vi "Abadines_Server2.vi"() -> ()   [LabVIEW 2013]
uses:
  <vilib>/NXT/Block Support/NXT_MessageMailbox.ctl
  <vilib>/NXT/Block Support/NXT_InputPort.ctl
  <vilib>/NXT/Dual Mode Library/BT/BlueTooth_Write_Num.vi
  <vilib>/NXT/Subs/MotorOutput.ctl
  <vilib>/NXT/Block Support/NXT_OutputPort.ctl
  <vilib>/NXT/LegoClasses/BrickReference/BrickReference.lvclass
  <vilib>/NXT/Subs/LVHSConnector.ctl
  <vilib>/NXT/NXTIO Xnodes/NXTIONodeSubVIs/NXTStopMotors.vi
  <vilib>/NXT/NXTIO Xnodes/NXTIOXNode/NXTIO.xnode
  <vilib>/NXT/NXTIO Xnodes/AddressXNode/NXTIOAddress.xnode
  <vilib>/NXT/Dual Mode Library/Sound/PlayRedPianoFile.vi
panel:
  out "Blue Line":i16
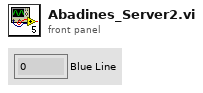
[diagram p1: front panel]
types:
  T1 = typedef "LVHSConnector.ctl" = refnum<class "BrickReference.lvclass">
  T2 = typedef "NXT_InputPort.ctl" = u32
  T3 = typedef "NXT_MessageMailbox.ctl" = u8
  T4 = typedef "NXT_OutputPort.ctl" = u8
  T5 = typedef "MotorOutput.ctl" = u8
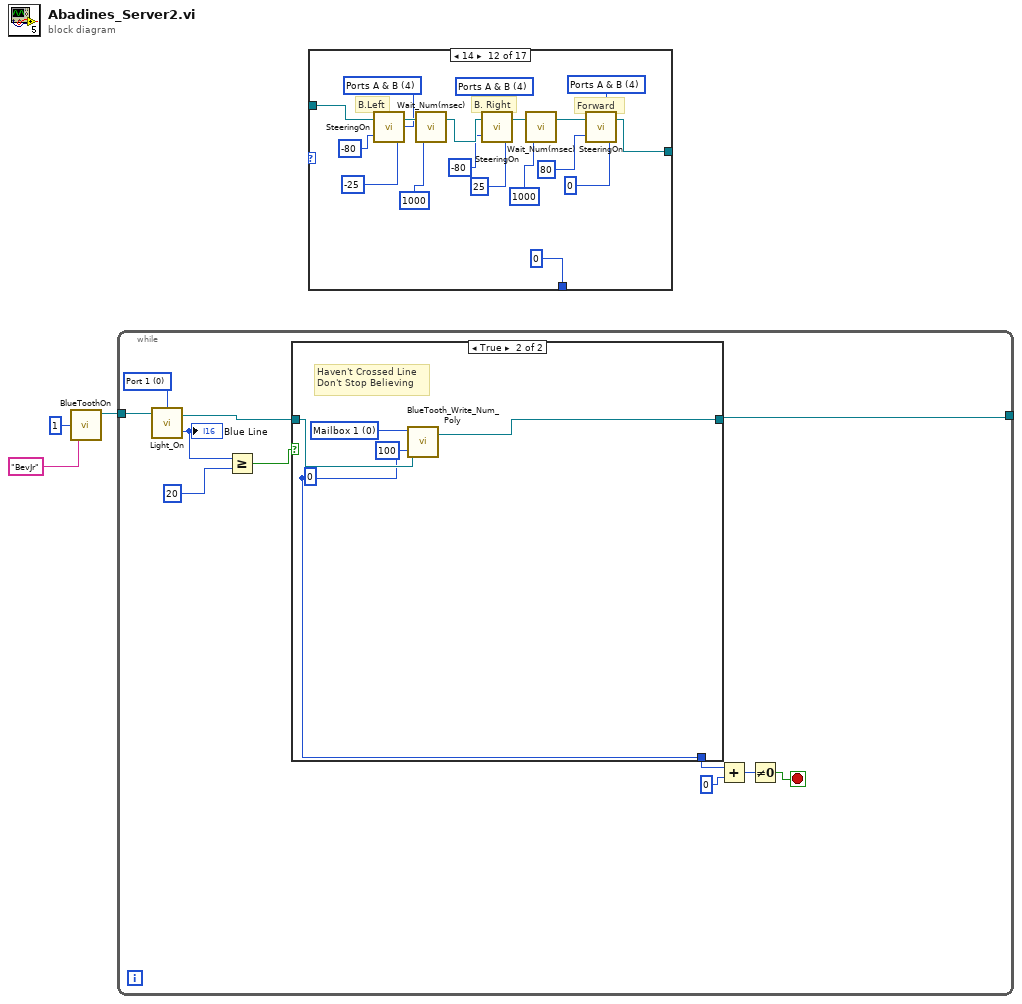
[diagram p0: block diagram]
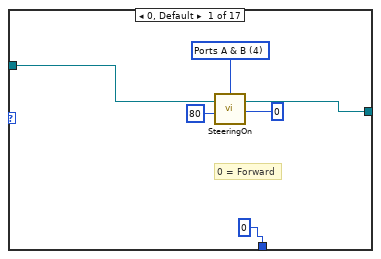
[diagram p2: hidden frame]
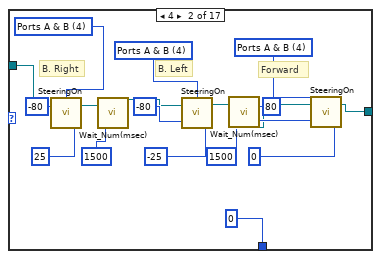
[diagram p3: hidden frame]
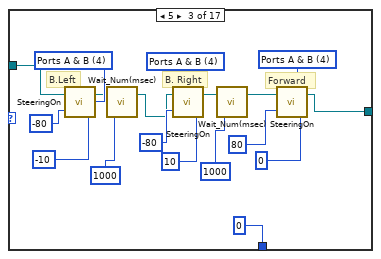
[diagram p4: hidden frame]
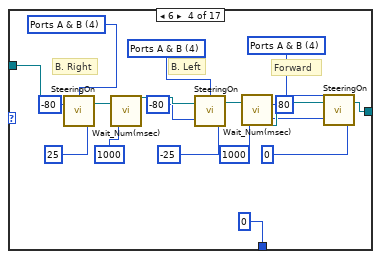
[diagram p5: hidden frame]
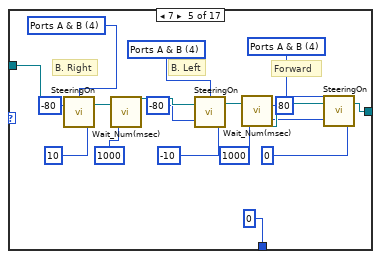
[diagram p6: hidden frame]
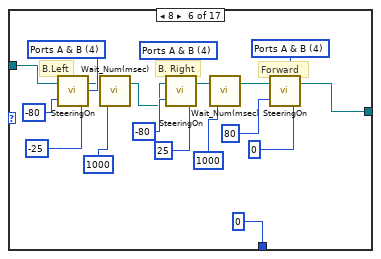
[diagram p7: hidden frame]
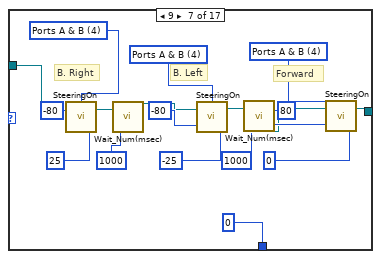
[diagram p8: hidden frame]
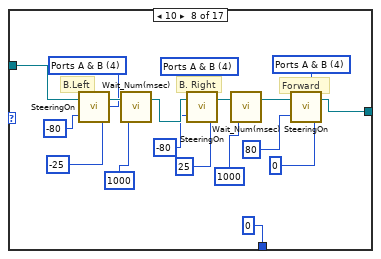
[diagram p9: hidden frame]
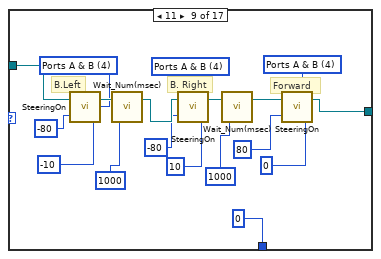
[diagram p10: hidden frame]
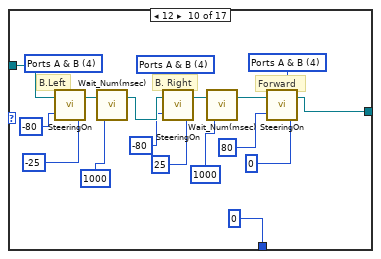
[diagram p11: hidden frame]
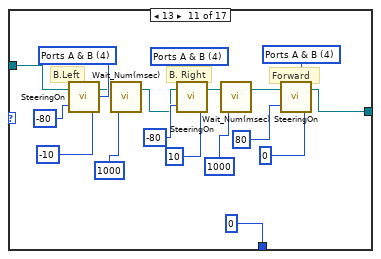
[diagram p12: hidden frame]
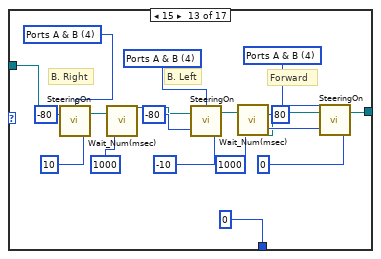
[diagram p13: hidden frame]
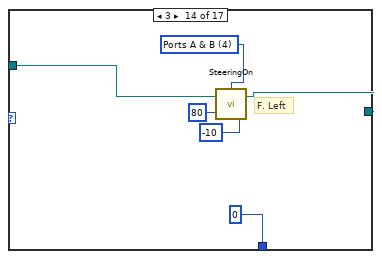
[diagram p14: hidden frame]
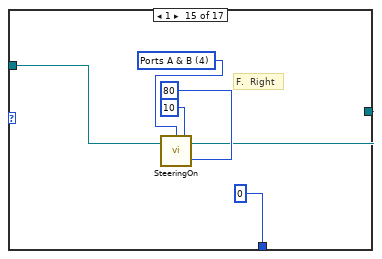
[diagram p15: hidden frame]
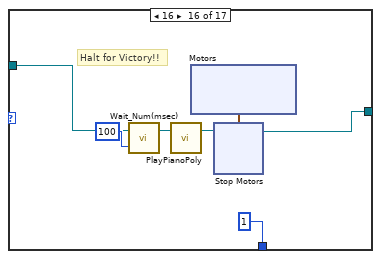
[diagram p16: hidden frame]
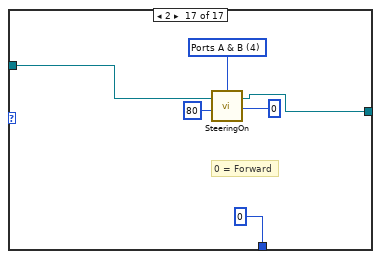
[diagram p17: hidden frame]
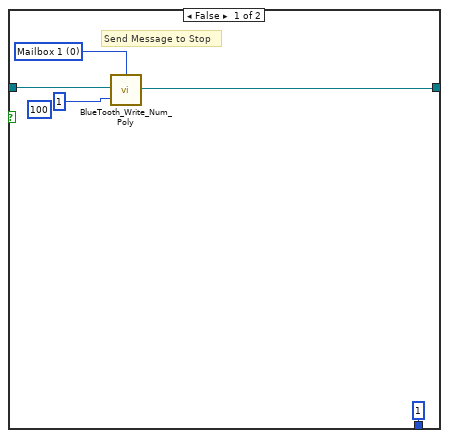
[diagram p18: hidden frame]
diagram:
  n1 = call "BlueToothOn.vi"("Connection"=u8 1, "Partner Name"="BevJr") -> ("NXT/EV3 2"=w2:T1)  [unwired: 1 in, 3 out]
  n2 = while {
    tunnel: w2 -> [w15]
    tunnel: [w9] -> _
    stop <- w5 stop-if-true
    w14 = T2 0 items=["Port 1", "Port 2", "Port 3", "Port 4"] ("Port (Port 3)")
    n3 = call <vilib>:"Light_On.vi"("NXT/EV3"=w15, "Port (Port 3)"=w14) -> ("Scaled Value"=w13:i16, "NXT/EV3"=w10:T1)  [unwired: 1 in]
    "Blue Line" <- w13
    n4 = Greater Or Equal?(x=w13, y=i16 20) -> (x >= y?=w11:bool)
    n5 = case shown="True" w11 {
      tunnel: w10 -> [w18 w23]
      tunnel: [w16 w22] -> w9
      tunnel: [1 w21] -> w8
      frame False {
        (unwired) u16 100 ("Tone (440 Hz)")
        w19 = T3 0 items=["Mailbox 1", "Mailbox 2", "Mailbox 3", "Mailbox 4", "Mailbox 5", "Mailbox 6", "Mailbox 7", "Mailbox 8", "Mailbox 9", "Mailbox 10"] ("Mailbox")
        # "Send Message to Stop"
        n6 = call-poly <vilib>:"BlueTooth_Write_Num_Poly.vi"("Message"=1, "NXT/EV3"=w18, "Mailbox"=w19) -> ("NXT/EV3"=w16:T1)  [unwired: 1 in]
      }
      frame True {
        (unwired) u16 100 ("Tone (440 Hz)")
        w24 = T3 0 items=["Mailbox 1", "Mailbox 2", "Mailbox 3", "Mailbox 4", "Mailbox 5", "Mailbox 6", "Mailbox 7", "Mailbox 8", "Mailbox 9", "Mailbox 10"] ("Mailbox")
        w21 = 0 ("Message")
        # "Haven't Crossed Line\nDon't Stop Believing"
        n7 = call-poly <vilib>:"BlueTooth_Write_Num_Poly.vi"("Message"=w21, "NXT/EV3"=w23, "Mailbox"=w24) -> ("NXT/EV3"=w22:T1)  [unwired: 1 in]
      }
    }
    n8 = Add(x=w8, y=0) -> (x+y=w6:i32)
    n9 = Not Equal To 0?(x=w6) -> (x != 0?=w5:bool)
  }
  n10 = case shown="14" {
    selector: _ -> [_ _ _ _ _ _ _ _ _ _ _ _ _ _ _ _ _]
    tunnel: _ -> [w28 w42 w51 w69 w87 w114 w123 w141 w159 w177 w194 w212 w231 w249 w255 w260 w274]
    tunnel: [w27 w41 w50 w68 w86 w113 w122 w140 w158 w176 w193 w211 w230 w248 w254 w261 w273] -> w1
    tunnel: [0 ("y") 0 ("y") 0 ("y") 0 ("y") 0 ("y") 0 ("y") 0 ("y") 0 ("y") 0 ("y") 0 ("y") 0 ("y") 0 ("y") 0 ("y") 0 ("y") 0 1 0 ("y")] -> _
    frame 0, Default {
      w26 = T5 4 items=["Port A"=0, "Port B"=1, "Port C"=2, "Ports A & B"=4, "Ports A & C"=5, "Ports B & C"=6, "All Ports"=3] ("Output Ports (A & B) 5")
      # "0 = Forward"
      n11 = call <vilib>:"SteeringOn.vi"("Power (75)"=80, "Steering (100)"=0, "NXT/EV3"=w28, "Output Ports (A & B)"=w26) -> ("NXT/EV3"=w27:T1)
    }
    frame 4 {
      w38 = T5 4 items=["Port A"=0, "Port B"=1, "Port C"=2, "Ports A & B"=4, "Ports A & C"=5, "Ports B & C"=6, "All Ports"=3] ("Output Ports (A & B) 15")
      w39 = T5 4 items=["Port A"=0, "Port B"=1, "Port C"=2, "Ports A & B"=4, "Ports A & C"=5, "Ports B & C"=6, "All Ports"=3] ("Output Port (All Ports) 6")
      w40 = T5 4 items=["Port A"=0, "Port B"=1, "Port C"=2, "Ports A & B"=4, "Ports A & C"=5, "Ports B & C"=6, "All Ports"=3] ("Output Ports (A & B) 16")
      # "Forward"
      # "B. Left"
      # "B. Right"
      n12 = call <vilib>:"SteeringOn.vi"("Power (75)"=-80, "Steering (100)"=25, "NXT/EV3"=w42, "Output Ports (A & B)"=w40) -> ("NXT/EV3"=w37:T1)
      n13 = call <vilib>:"Wait_Num(msec).vi"("Time (100 msec)"=u32 1500, "NXT/EV3"=w37) -> ("NXT/EV3"=w36:T1)  [unwired: 2 in]
      n14 = call <vilib>:"SteeringOn.vi"("Power (75)"=-80, "Steering (100)"=-25, "NXT/EV3"=w36, "Output Ports (A & B)"=w39) -> ("NXT/EV3"=w35:T1)
      n15 = call <vilib>:"Wait_Num(msec).vi"("Time (100 msec)"=u32 1500, "NXT/EV3"=w35) -> ("NXT/EV3"=w34:T1)  [unwired: 2 in]
      n16 = call <vilib>:"SteeringOn.vi"("Power (75)"=80, "Steering (100)"=0, "NXT/EV3"=w34, "Output Ports (A & B)"=w38) -> ("NXT/EV3"=w41:T1)
    }
    frame 5 {
      w58 = T5 4 items=["Port A"=0, "Port B"=1, "Port C"=2, "Ports A & B"=4, "Ports A & C"=5, "Ports B & C"=6, "All Ports"=3] ("Output Ports (A & B) 21")
      w59 = T5 4 items=["Port A"=0, "Port B"=1, "Port C"=2, "Ports A & B"=4, "Ports A & C"=5, "Ports B & C"=6, "All Ports"=3] ("Output Port (All Ports) 9")
      w60 = T5 4 items=["Port A"=0, "Port B"=1, "Port C"=2, "Ports A & B"=4, "Ports A & C"=5, "Ports B & C"=6, "All Ports"=3] ("Output Ports (A & B) 22")
      # "Forward"
      # "B. Right"
      # "B.Left"
      n17 = call <vilib>:"SteeringOn.vi"("Power (75)"=-80, "Steering (100)"=-10, "NXT/EV3"=w51, "Output Ports (A & B)"=w60) -> ("NXT/EV3"=w56:T1)
      n18 = call <vilib>:"Wait_Num(msec).vi"("Time (100 msec)"=u32 1000, "NXT/EV3"=w56) -> ("NXT/EV3"=w55:T1)  [unwired: 2 in]
      n19 = call <vilib>:"SteeringOn.vi"("Power (75)"=-80, "Steering (100)"=10, "NXT/EV3"=w55, "Output Ports (A & B)"=w59) -> ("NXT/EV3"=w53:T1)
      n20 = call <vilib>:"Wait_Num(msec).vi"("Time (100 msec)"=u32 1000, "NXT/EV3"=w53) -> ("NXT/EV3"=w52:T1)  [unwired: 2 in]
      n21 = call <vilib>:"SteeringOn.vi"("Power (75)"=80, "Steering (100)"=0, "NXT/EV3"=w52, "Output Ports (A & B)"=w58) -> ("NXT/EV3"=w50:T1)
    }
    frame 6 {
      w78 = T5 4 items=["Port A"=0, "Port B"=1, "Port C"=2, "Ports A & B"=4, "Ports A & C"=5, "Ports B & C"=6, "All Ports"=3] ("Output Ports (A & B) 15")
      w77 = T5 4 items=["Port A"=0, "Port B"=1, "Port C"=2, "Ports A & B"=4, "Ports A & C"=5, "Ports B & C"=6, "All Ports"=3] ("Output Port (All Ports) 6")
      w76 = T5 4 items=["Port A"=0, "Port B"=1, "Port C"=2, "Ports A & B"=4, "Ports A & C"=5, "Ports B & C"=6, "All Ports"=3] ("Output Ports (A & B) 16")
      # "Forward"
      # "B. Left"
      # "B. Right"
      n22 = call <vilib>:"SteeringOn.vi"("Power (75)"=-80, "Steering (100)"=25, "NXT/EV3"=w69, "Output Ports (A & B)"=w76) -> ("NXT/EV3"=w79:T1)
      n23 = call <vilib>:"Wait_Num(msec).vi"("Time (100 msec)"=u32 1000, "NXT/EV3"=w79) -> ("NXT/EV3"=w80:T1)  [unwired: 2 in]
      n24 = call <vilib>:"SteeringOn.vi"("Power (75)"=-80, "Steering (100)"=-25, "NXT/EV3"=w80, "Output Ports (A & B)"=w77) -> ("NXT/EV3"=w81:T1)
      n25 = call <vilib>:"Wait_Num(msec).vi"("Time (100 msec)"=u32 1000, "NXT/EV3"=w81) -> ("NXT/EV3"=w82:T1)  [unwired: 2 in]
      n26 = call <vilib>:"SteeringOn.vi"("Power (75)"=80, "Steering (100)"=0, "NXT/EV3"=w82, "Output Ports (A & B)"=w78) -> ("NXT/EV3"=w68:T1)
    }
    frame 7 {
      w96 = T5 4 items=["Port A"=0, "Port B"=1, "Port C"=2, "Ports A & B"=4, "Ports A & C"=5, "Ports B & C"=6, "All Ports"=3] ("Output Ports (A & B) 15")
      w95 = T5 4 items=["Port A"=0, "Port B"=1, "Port C"=2, "Ports A & B"=4, "Ports A & C"=5, "Ports B & C"=6, "All Ports"=3] ("Output Port (All Ports) 6")
      w94 = T5 4 items=["Port A"=0, "Port B"=1, "Port C"=2, "Ports A & B"=4, "Ports A & C"=5, "Ports B & C"=6, "All Ports"=3] ("Output Ports (A & B) 16")
      # "Forward"
      # "B. Left"
      # "B. Right"
      n27 = call <vilib>:"SteeringOn.vi"("Power (75)"=-80, "Steering (100)"=10, "NXT/EV3"=w87, "Output Ports (A & B)"=w94) -> ("NXT/EV3"=w97:T1)
      n28 = call <vilib>:"Wait_Num(msec).vi"("Time (100 msec)"=u32 1000, "NXT/EV3"=w97) -> ("NXT/EV3"=w98:T1)  [unwired: 2 in]
      n29 = call <vilib>:"SteeringOn.vi"("Power (75)"=-80, "Steering (100)"=-10, "NXT/EV3"=w98, "Output Ports (A & B)"=w95) -> ("NXT/EV3"=w99:T1)
      n30 = call <vilib>:"Wait_Num(msec).vi"("Time (100 msec)"=u32 1000, "NXT/EV3"=w99) -> ("NXT/EV3"=w100:T1)  [unwired: 2 in]
      n31 = call <vilib>:"SteeringOn.vi"("Power (75)"=80, "Steering (100)"=0, "NXT/EV3"=w100, "Output Ports (A & B)"=w96) -> ("NXT/EV3"=w86:T1)
    }
    frame 8 {
      w110 = T5 4 items=["Port A"=0, "Port B"=1, "Port C"=2, "Ports A & B"=4, "Ports A & C"=5, "Ports B & C"=6, "All Ports"=3] ("Output Ports (A & B) 21")
      w111 = T5 4 items=["Port A"=0, "Port B"=1, "Port C"=2, "Ports A & B"=4, "Ports A & C"=5, "Ports B & C"=6, "All Ports"=3] ("Output Port (All Ports) 9")
      w112 = T5 4 items=["Port A"=0, "Port B"=1, "Port C"=2, "Ports A & B"=4, "Ports A & C"=5, "Ports B & C"=6, "All Ports"=3] ("Output Ports (A & B) 22")
      # "Forward"
      # "B. Right"
      # "B.Left"
      n32 = call <vilib>:"SteeringOn.vi"("Power (75)"=-80, "Steering (100)"=-25, "NXT/EV3"=w114, "Output Ports (A & B)"=w112) -> ("NXT/EV3"=w108:T1)
      n33 = call <vilib>:"Wait_Num(msec).vi"("Time (100 msec)"=u32 1000, "NXT/EV3"=w108) -> ("NXT/EV3"=w107:T1)  [unwired: 2 in]
      n34 = call <vilib>:"SteeringOn.vi"("Power (75)"=-80, "Steering (100)"=25, "NXT/EV3"=w107, "Output Ports (A & B)"=w111) -> ("NXT/EV3"=w105:T1)
      n35 = call <vilib>:"Wait_Num(msec).vi"("Time (100 msec)"=u32 1000, "NXT/EV3"=w105) -> ("NXT/EV3"=w104:T1)  [unwired: 2 in]
      n36 = call <vilib>:"SteeringOn.vi"("Power (75)"=80, "Steering (100)"=0, "NXT/EV3"=w104, "Output Ports (A & B)"=w110) -> ("NXT/EV3"=w113:T1)
    }
    frame 9 {
      w130 = T5 4 items=["Port A"=0, "Port B"=1, "Port C"=2, "Ports A & B"=4, "Ports A & C"=5, "Ports B & C"=6, "All Ports"=3] ("Output Ports (A & B) 15")
      w131 = T5 4 items=["Port A"=0, "Port B"=1, "Port C"=2, "Ports A & B"=4, "Ports A & C"=5, "Ports B & C"=6, "All Ports"=3] ("Output Port (All Ports) 6")
      w132 = T5 4 items=["Port A"=0, "Port B"=1, "Port C"=2, "Ports A & B"=4, "Ports A & C"=5, "Ports B & C"=6, "All Ports"=3] ("Output Ports (A & B) 16")
      # "Forward"
      # "B. Left"
      # "B. Right"
      n37 = call <vilib>:"SteeringOn.vi"("Power (75)"=-80, "Steering (100)"=25, "NXT/EV3"=w123, "Output Ports (A & B)"=w132) -> ("NXT/EV3"=w129:T1)
      n38 = call <vilib>:"Wait_Num(msec).vi"("Time (100 msec)"=u32 1000, "NXT/EV3"=w129) -> ("NXT/EV3"=w128:T1)  [unwired: 2 in]
      n39 = call <vilib>:"SteeringOn.vi"("Power (75)"=-80, "Steering (100)"=-25, "NXT/EV3"=w128, "Output Ports (A & B)"=w131) -> ("NXT/EV3"=w127:T1)
      n40 = call <vilib>:"Wait_Num(msec).vi"("Time (100 msec)"=u32 1000, "NXT/EV3"=w127) -> ("NXT/EV3"=w126:T1)  [unwired: 2 in]
      n41 = call <vilib>:"SteeringOn.vi"("Power (75)"=80, "Steering (100)"=0, "NXT/EV3"=w126, "Output Ports (A & B)"=w130) -> ("NXT/EV3"=w122:T1)
    }
    frame 10 {
      w150 = T5 4 items=["Port A"=0, "Port B"=1, "Port C"=2, "Ports A & B"=4, "Ports A & C"=5, "Ports B & C"=6, "All Ports"=3] ("Output Ports (A & B) 21")
      w149 = T5 4 items=["Port A"=0, "Port B"=1, "Port C"=2, "Ports A & B"=4, "Ports A & C"=5, "Ports B & C"=6, "All Ports"=3] ("Output Port (All Ports) 9")
      w148 = T5 4 items=["Port A"=0, "Port B"=1, "Port C"=2, "Ports A & B"=4, "Ports A & C"=5, "Ports B & C"=6, "All Ports"=3] ("Output Ports (A & B) 22")
      # "Forward"
      # "B. Right"
      # "B.Left"
      n42 = call <vilib>:"SteeringOn.vi"("Power (75)"=-80, "Steering (100)"=-25, "NXT/EV3"=w141, "Output Ports (A & B)"=w148) -> ("NXT/EV3"=w152:T1)
      n43 = call <vilib>:"Wait_Num(msec).vi"("Time (100 msec)"=u32 1000, "NXT/EV3"=w152) -> ("NXT/EV3"=w153:T1)  [unwired: 2 in]
      n44 = call <vilib>:"SteeringOn.vi"("Power (75)"=-80, "Steering (100)"=25, "NXT/EV3"=w153, "Output Ports (A & B)"=w149) -> ("NXT/EV3"=w155:T1)
      n45 = call <vilib>:"Wait_Num(msec).vi"("Time (100 msec)"=u32 1000, "NXT/EV3"=w155) -> ("NXT/EV3"=w156:T1)  [unwired: 2 in]
      n46 = call <vilib>:"SteeringOn.vi"("Power (75)"=80, "Steering (100)"=0, "NXT/EV3"=w156, "Output Ports (A & B)"=w150) -> ("NXT/EV3"=w140:T1)
    }
    frame 11 {
      w168 = T5 4 items=["Port A"=0, "Port B"=1, "Port C"=2, "Ports A & B"=4, "Ports A & C"=5, "Ports B & C"=6, "All Ports"=3] ("Output Ports (A & B) 21")
      w167 = T5 4 items=["Port A"=0, "Port B"=1, "Port C"=2, "Ports A & B"=4, "Ports A & C"=5, "Ports B & C"=6, "All Ports"=3] ("Output Port (All Ports) 9")
      w166 = T5 4 items=["Port A"=0, "Port B"=1, "Port C"=2, "Ports A & B"=4, "Ports A & C"=5, "Ports B & C"=6, "All Ports"=3] ("Output Ports (A & B) 22")
      # "Forward"
      # "B. Right"
      # "B.Left"
      n47 = call <vilib>:"SteeringOn.vi"("Power (75)"=-80, "Steering (100)"=-10, "NXT/EV3"=w159, "Output Ports (A & B)"=w166) -> ("NXT/EV3"=w170:T1)
      n48 = call <vilib>:"Wait_Num(msec).vi"("Time (100 msec)"=u32 1000, "NXT/EV3"=w170) -> ("NXT/EV3"=w171:T1)  [unwired: 2 in]
      n49 = call <vilib>:"SteeringOn.vi"("Power (75)"=-80, "Steering (100)"=10, "NXT/EV3"=w171, "Output Ports (A & B)"=w167) -> ("NXT/EV3"=w173:T1)
      n50 = call <vilib>:"Wait_Num(msec).vi"("Time (100 msec)"=u32 1000, "NXT/EV3"=w173) -> ("NXT/EV3"=w174:T1)  [unwired: 2 in]
      n51 = call <vilib>:"SteeringOn.vi"("Power (75)"=80, "Steering (100)"=0, "NXT/EV3"=w174, "Output Ports (A & B)"=w168) -> ("NXT/EV3"=w158:T1)
    }
    frame 12 {
      w185 = T5 4 items=["Port A"=0, "Port B"=1, "Port C"=2, "Ports A & B"=4, "Ports A & C"=5, "Ports B & C"=6, "All Ports"=3] ("Output Ports (A & B) 21")
      w184 = T5 4 items=["Port A"=0, "Port B"=1, "Port C"=2, "Ports A & B"=4, "Ports A & C"=5, "Ports B & C"=6, "All Ports"=3] ("Output Port (All Ports) 9")
      (unwired) T5 4 items=["Port A"=0, "Port B"=1, "Port C"=2, "Ports A & B"=4, "Ports A & C"=5, "Ports B & C"=6, "All Ports"=3] ("Output Ports (A & B) 22")
      # "Forward"
      # "B. Right"
      # "B.Left"
      n52 = call <vilib>:"SteeringOn.vi"("Power (75)"=-80, "Steering (100)"=-25, "NXT/EV3"=w177) -> ("NXT/EV3"=w187:T1)  [unwired: 1 in]
      n53 = call <vilib>:"Wait_Num(msec).vi"("Time (100 msec)"=u32 1000, "NXT/EV3"=w187) -> ("NXT/EV3"=w188:T1)  [unwired: 2 in]
      n54 = call <vilib>:"SteeringOn.vi"("Power (75)"=-80, "Steering (100)"=25, "NXT/EV3"=w188, "Output Ports (A & B)"=w184) -> ("NXT/EV3"=w190:T1)
      n55 = call <vilib>:"Wait_Num(msec).vi"("Time (100 msec)"=u32 1000, "NXT/EV3"=w190) -> ("NXT/EV3"=w191:T1)  [unwired: 2 in]
      n56 = call <vilib>:"SteeringOn.vi"("Power (75)"=80, "Steering (100)"=0, "NXT/EV3"=w191, "Output Ports (A & B)"=w185) -> ("NXT/EV3"=w176:T1)
    }
    frame 13 {
      w201 = T5 4 items=["Port A"=0, "Port B"=1, "Port C"=2, "Ports A & B"=4, "Ports A & C"=5, "Ports B & C"=6, "All Ports"=3] ("Output Ports (A & B) 21")
      w202 = T5 4 items=["Port A"=0, "Port B"=1, "Port C"=2, "Ports A & B"=4, "Ports A & C"=5, "Ports B & C"=6, "All Ports"=3] ("Output Port (All Ports) 9")
      w203 = T5 4 items=["Port A"=0, "Port B"=1, "Port C"=2, "Ports A & B"=4, "Ports A & C"=5, "Ports B & C"=6, "All Ports"=3] ("Output Ports (A & B) 22")
      # "Forward"
      # "B. Right"
      # "B.Left"
      n57 = call <vilib>:"SteeringOn.vi"("Power (75)"=-80, "Steering (100)"=-10, "NXT/EV3"=w194, "Output Ports (A & B)"=w203) -> ("NXT/EV3"=w199:T1)
      n58 = call <vilib>:"Wait_Num(msec).vi"("Time (100 msec)"=u32 1000, "NXT/EV3"=w199) -> ("NXT/EV3"=w198:T1)  [unwired: 2 in]
      n59 = call <vilib>:"SteeringOn.vi"("Power (75)"=-80, "Steering (100)"=10, "NXT/EV3"=w198, "Output Ports (A & B)"=w202) -> ("NXT/EV3"=w196:T1)
      n60 = call <vilib>:"Wait_Num(msec).vi"("Time (100 msec)"=u32 1000, "NXT/EV3"=w196) -> ("NXT/EV3"=w195:T1)  [unwired: 2 in]
      n61 = call <vilib>:"SteeringOn.vi"("Power (75)"=80, "Steering (100)"=0, "NXT/EV3"=w195, "Output Ports (A & B)"=w201) -> ("NXT/EV3"=w193:T1)
    }
    frame 14 {
      w221 = T5 4 items=["Port A"=0, "Port B"=1, "Port C"=2, "Ports A & B"=4, "Ports A & C"=5, "Ports B & C"=6, "All Ports"=3] ("Output Ports (A & B) 21")
      w220 = T5 4 items=["Port A"=0, "Port B"=1, "Port C"=2, "Ports A & B"=4, "Ports A & C"=5, "Ports B & C"=6, "All Ports"=3] ("Output Port (All Ports) 9")
      w219 = T5 4 items=["Port A"=0, "Port B"=1, "Port C"=2, "Ports A & B"=4, "Ports A & C"=5, "Ports B & C"=6, "All Ports"=3] ("Output Ports (A & B) 22")
      # "Forward"
      # "B. Right"
      # "B.Left"
      n62 = call <vilib>:"SteeringOn.vi"("Power (75)"=-80, "Steering (100)"=-25, "NXT/EV3"=w212, "Output Ports (A & B)"=w219) -> ("NXT/EV3"=w223:T1)
      n63 = call <vilib>:"Wait_Num(msec).vi"("Time (100 msec)"=u32 1000, "NXT/EV3"=w223) -> ("NXT/EV3"=w224:T1)  [unwired: 2 in]
      n64 = call <vilib>:"SteeringOn.vi"("Power (75)"=-80, "Steering (100)"=25, "NXT/EV3"=w224, "Output Ports (A & B)"=w220) -> ("NXT/EV3"=w226:T1)
      n65 = call <vilib>:"Wait_Num(msec).vi"("Time (100 msec)"=u32 1000, "NXT/EV3"=w226) -> ("NXT/EV3"=w227:T1)  [unwired: 2 in]
      n66 = call <vilib>:"SteeringOn.vi"("Power (75)"=80, "Steering (100)"=0, "NXT/EV3"=w227, "Output Ports (A & B)"=w221) -> ("NXT/EV3"=w211:T1)
    }
    frame 15 {
      w238 = T5 4 items=["Port A"=0, "Port B"=1, "Port C"=2, "Ports A & B"=4, "Ports A & C"=5, "Ports B & C"=6, "All Ports"=3] ("Output Ports (A & B) 15")
      w239 = T5 4 items=["Port A"=0, "Port B"=1, "Port C"=2, "Ports A & B"=4, "Ports A & C"=5, "Ports B & C"=6, "All Ports"=3] ("Output Port (All Ports) 6")
      w229 = T5 4 items=["Port A"=0, "Port B"=1, "Port C"=2, "Ports A & B"=4, "Ports A & C"=5, "Ports B & C"=6, "All Ports"=3] ("Output Ports (A & B) 16")
      # "Forward"
      # "B. Left"
      # "B. Right"
      n67 = call <vilib>:"SteeringOn.vi"("Power (75)"=-80, "Steering (100)"=10, "NXT/EV3"=w231, "Output Ports (A & B)"=w229) -> ("NXT/EV3"=w237:T1)
      n68 = call <vilib>:"Wait_Num(msec).vi"("Time (100 msec)"=u32 1000, "NXT/EV3"=w237) -> ("NXT/EV3"=w236:T1)  [unwired: 2 in]
      n69 = call <vilib>:"SteeringOn.vi"("Power (75)"=-80, "Steering (100)"=-10, "NXT/EV3"=w236, "Output Ports (A & B)"=w239) -> ("NXT/EV3"=w235:T1)
      n70 = call <vilib>:"Wait_Num(msec).vi"("Time (100 msec)"=u32 1000, "NXT/EV3"=w235) -> ("NXT/EV3"=w234:T1)  [unwired: 2 in]
      n71 = call <vilib>:"SteeringOn.vi"("Power (75)"=80, "Steering (100)"=0, "NXT/EV3"=w234, "Output Ports (A & B)"=w238) -> ("NXT/EV3"=w230:T1)
    }
    frame 3 {
      w247 = T5 4 items=["Port A"=0, "Port B"=1, "Port C"=2, "Ports A & B"=4, "Ports A & C"=5, "Ports B & C"=6, "All Ports"=3] ("Output Port (All Ports) 3")
      # "F. Left"
      n72 = call <vilib>:"SteeringOn.vi"("Power (75)"=80, "Steering (100)"=-10, "NXT/EV3"=w249, "Output Ports (A & B)"=w247) -> ("NXT/EV3"=w248:T1)
    }
    frame 1 {
      w253 = T5 4 items=["Port A"=0, "Port B"=1, "Port C"=2, "Ports A & B"=4, "Ports A & C"=5, "Ports B & C"=6, "All Ports"=3] ("Output Ports (A & B) 12")
      # "F.  Right"
      n73 = call <vilib>:"SteeringOn.vi"("Power (75)"=80, "Steering (100)"=10, "NXT/EV3"=w255, "Output Ports (A & B)"=w253) -> ("NXT/EV3"=w254:T1)
    }
    frame 16 {
      # "Halt for Victory!!"
      n74 = call <vilib>:"Wait_Num(msec).vi"("Time (100 msec)"=u32 100, "NXT/EV3"=w260) -> ("NXT/EV3"=w259:T1)  [unwired: 2 in]
      n75 = call-poly <vilib>:"PlayPianoPoly.vi"("NXT/EV3"=w259) -> ("NXT/EV3"=w258:T1)  [unwired: 3 in]
      n76 = xnode "Motors"() -> ("Motor"=w264:cluster{"Port":T4, "Port":T4})
      n77 = xnode "Stop Motors"("Motors"=w264, "NXT/EV3"=w258) -> ("NXT/EV3"=w261:T1)
    }
    frame 2 {
      w272 = T5 4 items=["Port A"=0, "Port B"=1, "Port C"=2, "Ports A & B"=4, "Ports A & C"=5, "Ports B & C"=6, "All Ports"=3] ("Output Ports (A & B) 10")
      # "0 = Forward"
      n78 = call <vilib>:"SteeringOn.vi"("Power (75)"=80, "Steering (100)"=0, "NXT/EV3"=w274, "Output Ports (A & B)"=w272) -> ("NXT/EV3"=w273:T1)
    }
  }
